vi "Analyse libreVNA.vi"() -> ()   [LabVIEW 2020]
uses:
  common/record_file_handler/VFH-VNA_File_Handler.lvlib
panel:
  out "Magnitude":cluster{"Frequency":dbl[], "S11_Real":dbl[]}[](graph)
  out "Z":cluster{"Frequency":dbl[], "S11_Real":dbl[]}[](graph)
  out "S11''":cluster{"Frequency":dbl[], "S11_Real":dbl[]}[](graph)
  out "S11'":cluster{"Frequency":dbl[], "S11_Real":dbl[]}[](graph)
  out "Array":string[](array[string])
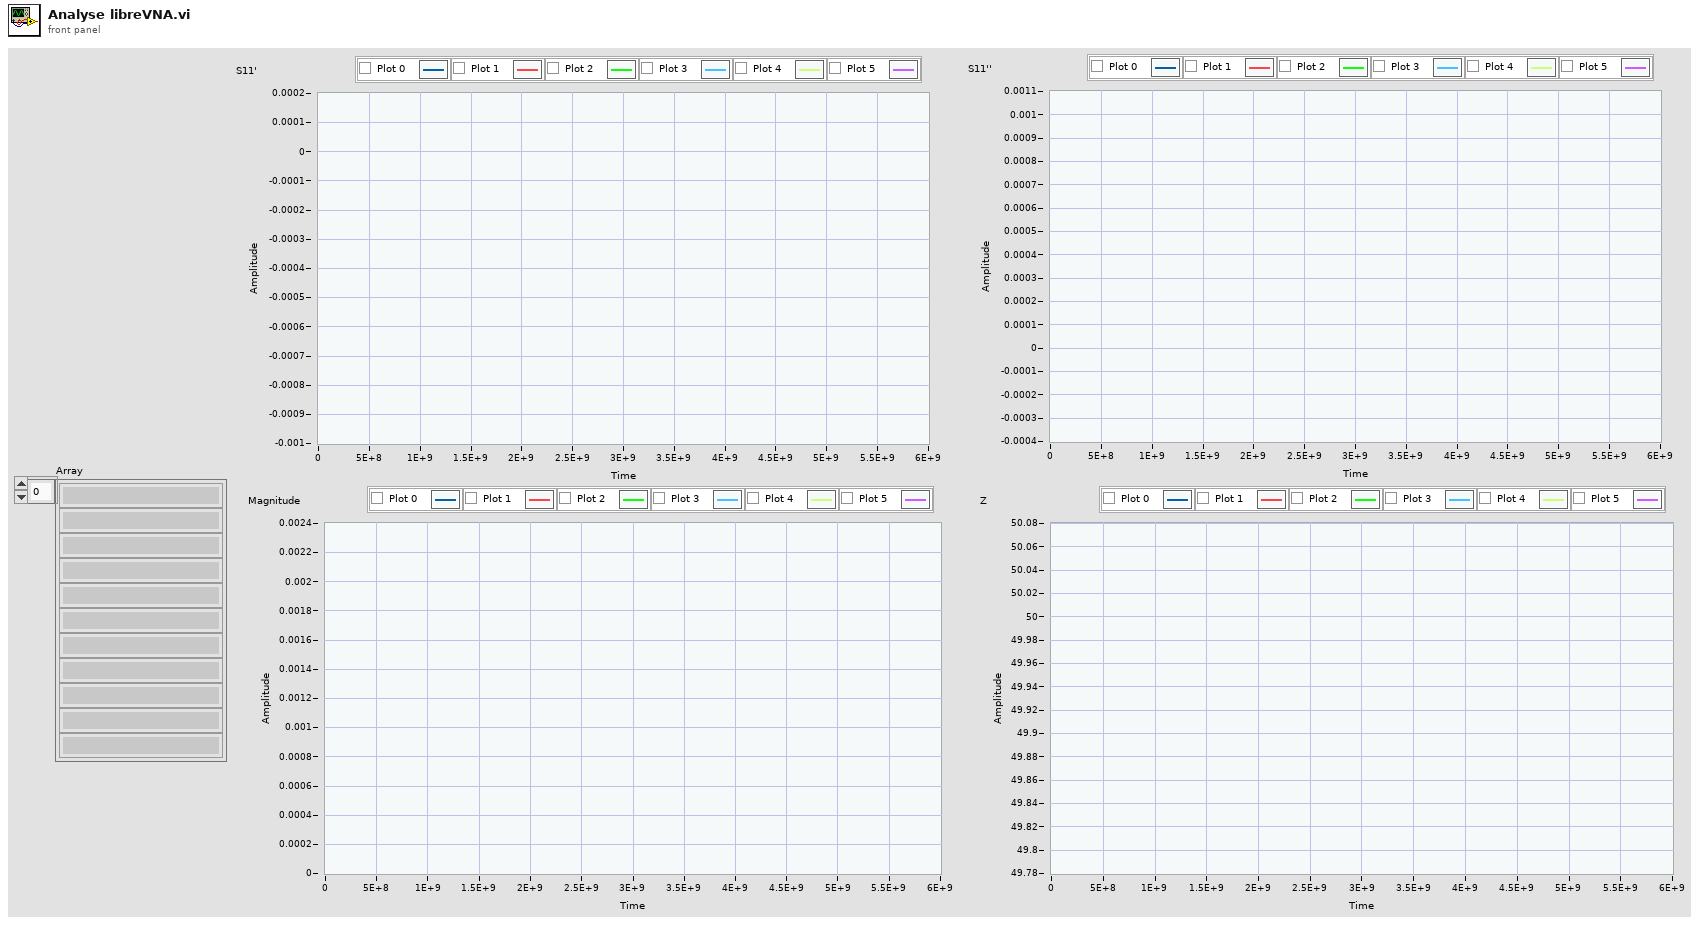
[diagram p1: front panel]
types:
  T1 = typedef "VFH-VNA_File_Handler.lvlib/VFH-file_cluster-NanoVNA.ctl" = cluster{"Frequency":dbl[], "S11_Real":dbl[], "S11_Imag":dbl[], "S21_Real":dbl[], "S21_Imag":dbl[], "S12_Real":dbl[], "S12_Imag":dbl[], "S22_Real":dbl[], "S22_Imag":dbl[]}
  T2 = cluster{"Loss":cluster{"Frequency":dbl[], "Array":dbl[]}, "Z Modulus":cluster{"Frequency":dbl[], "Array":dbl[]}, "Z'":cluster{"Frequency":dbl[], "Array":dbl[]}, "Z''":cluster{"Frequency":dbl[], "Array":dbl[]}}
  T3 = cluster{"S11'":cluster{"Frequency":dbl[], "S11_Real":dbl[]}, "S11''":cluster{"Frequency":dbl[], "S11_Real":dbl[]}, "Magnitude":cluster{"Frequency":dbl[], "Array":dbl[]}, "Eta":cluster{"Frequency":dbl[], "Array":dbl[]}, "Phase":cluster{"Frequency":dbl[], "Array":dbl[]}}
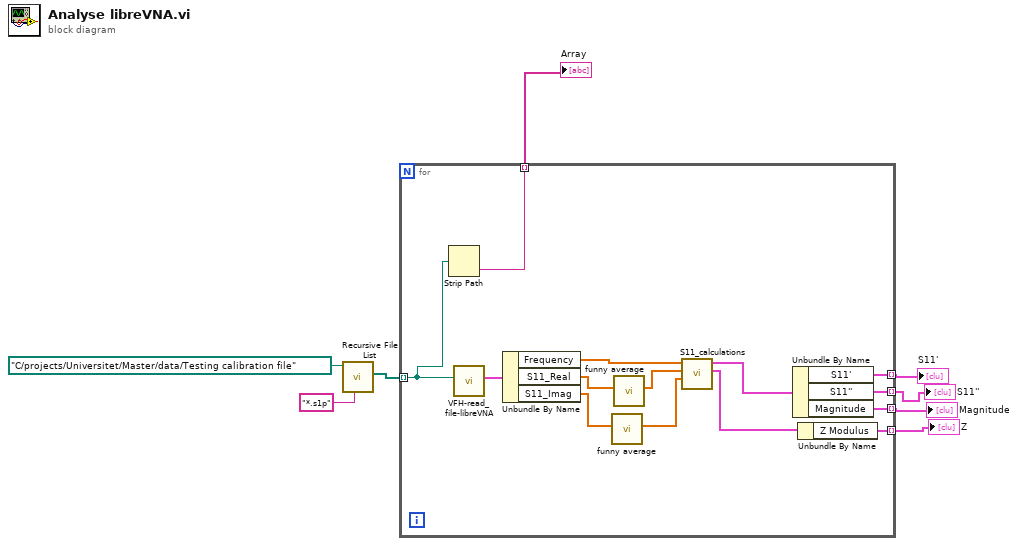
[diagram p0: block diagram]
diagram:
  n1 = call <vilib>:"Recursive File List.vi"("pattern"="*.s1p", "Folder Path"=path "C:/projects/Universitet/Master/data/Testing calibration file" ("base path")) -> ("All Files in Dir"=w7:path[])  [unwired: 5 in, 4 out]
  n2 = for {
    tunnel: w7 -> [w10] mode=indexing
    tunnel: [w19] -> w5 mode=indexing
    tunnel: [w18] -> w4 mode=indexing
    tunnel: [w17] -> w3 mode=indexing
    tunnel: [w16] -> w2 mode=indexing
    tunnel: [w11] -> w6 mode=indexing
    n3 = Strip Path(path=w10) -> (name=w11:string)  [unwired: 1 out]
    n4 = call "VFH-read_file-libreVNA.vi"("file path (dialog if empty)"=w10) -> ("output cluster"=w9:T1)  [unwired: 9 in, 1 out]
    n5 = Unbundle By Name(w9) -> ("Frequency"=w22:dbl[], "S11_Real"=w15:dbl[], "S11_Imag"=w13:dbl[])
    n6 = call "funny average.vi"("in"=w13) -> ("Out"=w12:dbl[])  [unwired: 10 in]
    n7 = call "funny average.vi"("in"=w15) -> ("Out"=w14:dbl[])  [unwired: 10 in]
    n8 = call "S11_calculations.vi"("S11_Imag"=w12, "S11_Real"=w14, "Frequency"=w22) -> ("Calc"=w20:T2, "Raw"=w21:T3)  [unwired: 6 in, 1 out]
    n9 = Unbundle By Name(w21) -> ("S11'"=w19:cluster{"Frequency":dbl[], "S11_Real":dbl[]}, "S11''"=w18:cluster{"Frequency":dbl[], "S11_Real":dbl[]}, "Magnitude"=w17:cluster{"Frequency":dbl[], "Array":dbl[]})
    n10 = Unbundle By Name(w20) -> ("Z Modulus"=w16:cluster{"Frequency":dbl[], "Array":dbl[]})
  }
  "Array" <- w6
  "S11'" <- w5
  "S11''" <- w4
  "Z" <- w2
  "Magnitude" <- w3
